vi "variable_steps_logic.vi"(2 "Num files":i32=1, 3 "Variable Steps":bool, 4 "Voltage 2":dbl, 5 "Voltage 1":dbl, 6 "iteration number":i32) -> (0 "Returned Voltage 2":dbl, 1 "Returned Voltage 1":dbl)   [LabVIEW 2016]
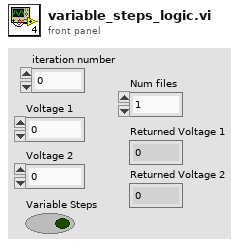
[diagram p1: front panel]
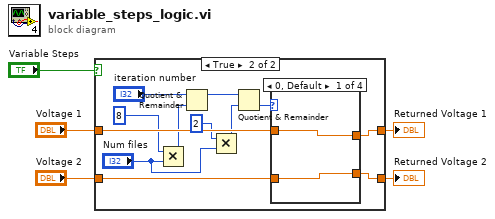
[diagram p0: block diagram]
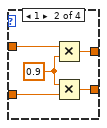
[diagram p3: hidden frame]
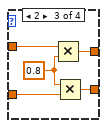
[diagram p4: hidden frame]
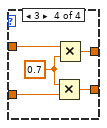
[diagram p5: hidden frame]
diagram:
  n1 = case shown="True" "Variable Steps" {
    tunnel: "Voltage 1" -> [w7 w17]
    tunnel: "Voltage 2" -> [w6 w15]
    tunnel: [w7 w18] -> w2
    tunnel: [w6 w16] -> w1
    frame False {
    }
    frame True {
      n2 = Multiply(x=8 ("y"), y="Num files") -> (x*y=w11:i32)
      n3 = Quotient & Remainder(x="iteration number", y=w11) -> (x-y*floor(x/y)=w14:i32)  [unwired: 1 out]
      n4 = Multiply(x=2 ("y"), y="Num files") -> (x*y=w8:i32)
      n5 = Quotient & Remainder(x=w14, y=w8) -> (floor(x/y)=w13:i32)  [unwired: 1 out]
      n6 = case shown="0, Default" w13 {
        tunnel: [w21 w25 w30 w35] -> w18
        tunnel: w17 -> [w21 w26 w31 w36]
        tunnel: [w20 w24 w29 w34] -> w16
        tunnel: w15 -> [w20 w23 w28 w33]
        frame 0, Default {
        }
        frame 1 {
          w22 = 0.9 ("y")
          n7 = Multiply(x=w26, y=w22) -> (x*y=w25:dbl)
          n8 = Multiply(x=w22, y=w23) -> (x*y=w24:dbl)
        }
        frame 2 {
          w27 = 0.8 ("y")
          n9 = Multiply(x=w31, y=w27) -> (x*y=w30:dbl)
          n10 = Multiply(x=w27, y=w28) -> (x*y=w29:dbl)
        }
        frame 3 {
          w32 = 0.7 ("y")
          n11 = Multiply(x=w32, y=w33) -> (x*y=w34:dbl)
          n12 = Multiply(x=w36, y=w32) -> (x*y=w35:dbl)
        }
      }
    }
  }
  "Returned Voltage 1" <- w2
  "Returned Voltage 2" <- w1
